vi "SetDev Scope Resource.vi"(8 "error in (no error)":errorcluster, 9 "Scope VISA Addr":refnum<visa-resource-name>, 10 "Simulated":bool, 11 "Actor_Scope in":refnum<class "Actor_Scope.lvclass">) -> (0 "error out":errorcluster, 3 "Actor_Scope out":refnum<class "Actor_Scope.lvclass">)   [LabVIEW 2020, in "Actor_Scope.lvlib" / "Actor_Scope.lvclass"]
uses:
  Actor_Scope.lvclass
  Actor_Scope.lvclass/Actor_Scope.ctl
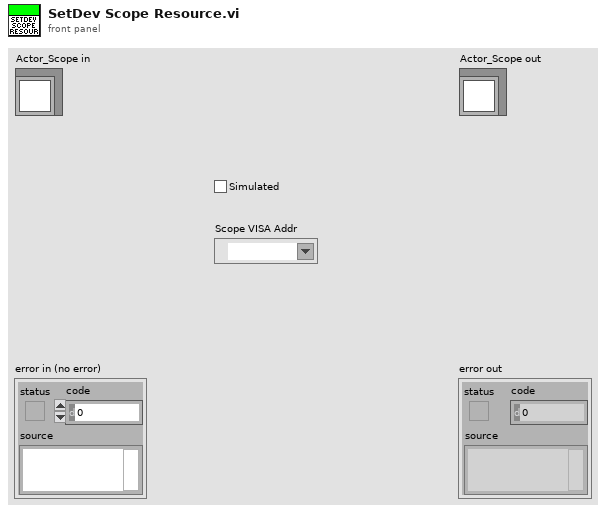
[diagram p1: front panel]
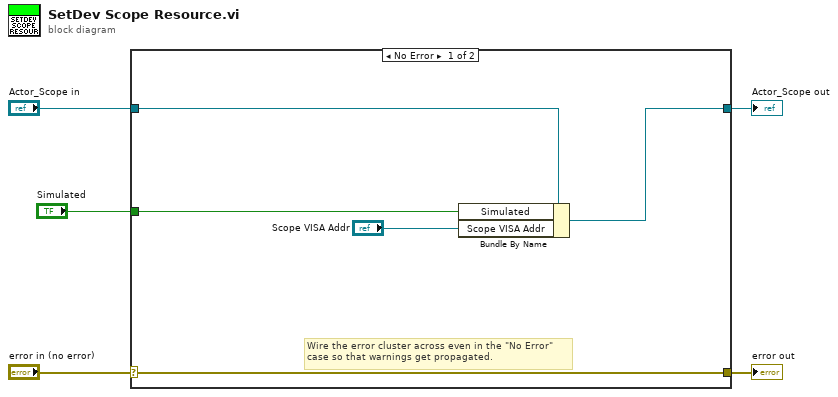
[diagram p0: block diagram]
diagram:
  n1 = case shown="No Error" "error in (no error)" {
    selector: "error in (no error)" -> [w10 w12]
    tunnel: [w10 w12] -> w4
    tunnel: [w6 w11] -> w2
    tunnel: "Actor_Scope in" -> [w7 w11]
    tunnel: "Simulated" -> [w8 _]
    frame No Error {
      # "Wire the error cluster across even in the \"No Error\"\ncase so that warnings get propagated."
      n2 = Bundle By Name(cluster=w7, "Simulated"=w8, "Scope VISA Addr"="Scope VISA Addr") -> (w6:refnum<class "Actor_Scope.lvclass">)
    }
    frame Error {
    }
  }
  "error out" <- w4
  "Actor_Scope out" <- w2
